vi "initialize assembly lists.vi"(4 "output dictionary":refnum<class "data dictionary.lvclass">, 6 "input dictionary":refnum<class "data dictionary.lvclass">, 8 "error in":errorcluster, 10 "EthernetIP configuration in":refnum<class "EthernetIP configuration.lvclass">, 11 "EthernetIP runtime in":refnum<class "EthernetIP runtime.lvclass">) -> (0 "error out":errorcluster, 3 "EthernetIP runtime out":refnum<class "EthernetIP runtime.lvclass">)   [LabVIEW 2013, in "EthernetIP runtime.lvclass"]
uses:
  EthernetIP runtime.lvclass
  configuration/EthernetIP configuration.lvclass
  <vilib>/NI/Tag Bus/dictionary/data dictionary.lvclass
  <vilib>/ethernetip/ethernetip.llb/ethernetip.ctl
  assembly data spec.ctl
  conversion specification.ctl
  <vilib>/NI/Tag Bus/tag/Data Type.ctl
  configuration/EthernetIP configuration.lvclass/EthernetIP configuration.ctl
  <vilib>/ethernetip/ethernetip.llb/EthernetIPAssemblyType.ctl
  channel/EthernetIP Channel.lvclass/EthernetIP Channel.ctl
  <vilib>/NI/Tag Bus/tag/tag descriptor.lvclass/tag descriptor.ctl
  <vilib>/NI/Tag Bus Module Framework/channel/TBM channel.lvclass/TBM channel.ctl
  EthernetIP runtime.lvclass/EthernetIP runtime.ctl
  channel/Read Instance ID.vi
  <vilib>/NI/Tag Bus/tag/read tag name.vi
  <vilib>/NI/Tag Bus Module Framework/channel/Read channel classification.vi
  <vilib>/NI/Tag Bus/tag/read data type.vi
  channel/Read byte index.vi
  configuration/Read assemblies.vi
  configuration/read eip channels.vi
  channel/EthernetIP Channel.lvclass
  <vilib>/NI/Tag Bus/tag/tag descriptor.lvclass
  <vilib>/ethernetip/ethernetip.lvlib
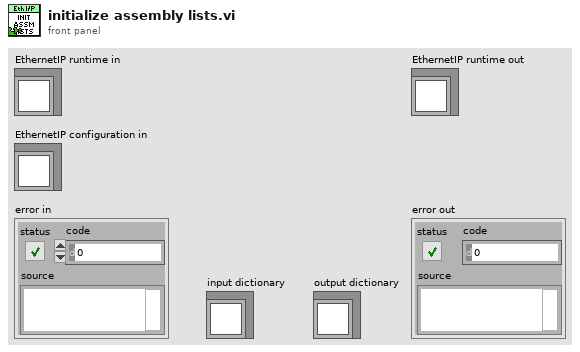
[diagram p1: front panel]
types:
  T1 = typedef "EthernetIP runtime.lvclass/assembly data spec.ctl" = cluster{"Instance ID":u32, "specification":T2[], "big endian?":bool}
  T2 = typedef "EthernetIP runtime.lvclass/conversion specification.ctl" = cluster{"data type":T3, "data index":i32, "byte index":i32, "subindex/len":i32}
  T3 = typedef "tag bus.lvlib/tag descriptor.lvclass/Data Type.ctl" = enum16{"Double", "Single", "I64", "I32", "I16", "I8", "U64", "U32", "U16", "U8", "Boolean", "String", "Array of Double", "Array of Single", "Array of I64", "Array of I32", "Array of I16", "Array of I8", "Array of U64", "Array of U32", "Array of U16", "Array of U8", "Array of Boolean", "Array of String"}
  T4 = typedef "ethernetip.lvlib/ethernetip.ctl" = refnum<k21>
  T5 = typedef "EthernetIP configuration.lvclass/assembly definition.ctl" = cluster{"name":string, "Instance ID":u32, "Type":T6, "Size (elements)":u32, "big endian?":bool, "data type":T3}
  T6 = typedef "EthernetIP configuration.lvclass/assembly type.ctl" = enum32{"Producing", "Consuming"}
  T7 = typedef "ethernetip.lvlib/EthernetIPAssemblyType.ctl" = enum16{"Producing", "Consuming", "Configuration"}
  T8 = typedef "TBM channel.lvclass/channel classification.ctl" = enum16{"input data", "output data", "processing parameter", "processing result"}
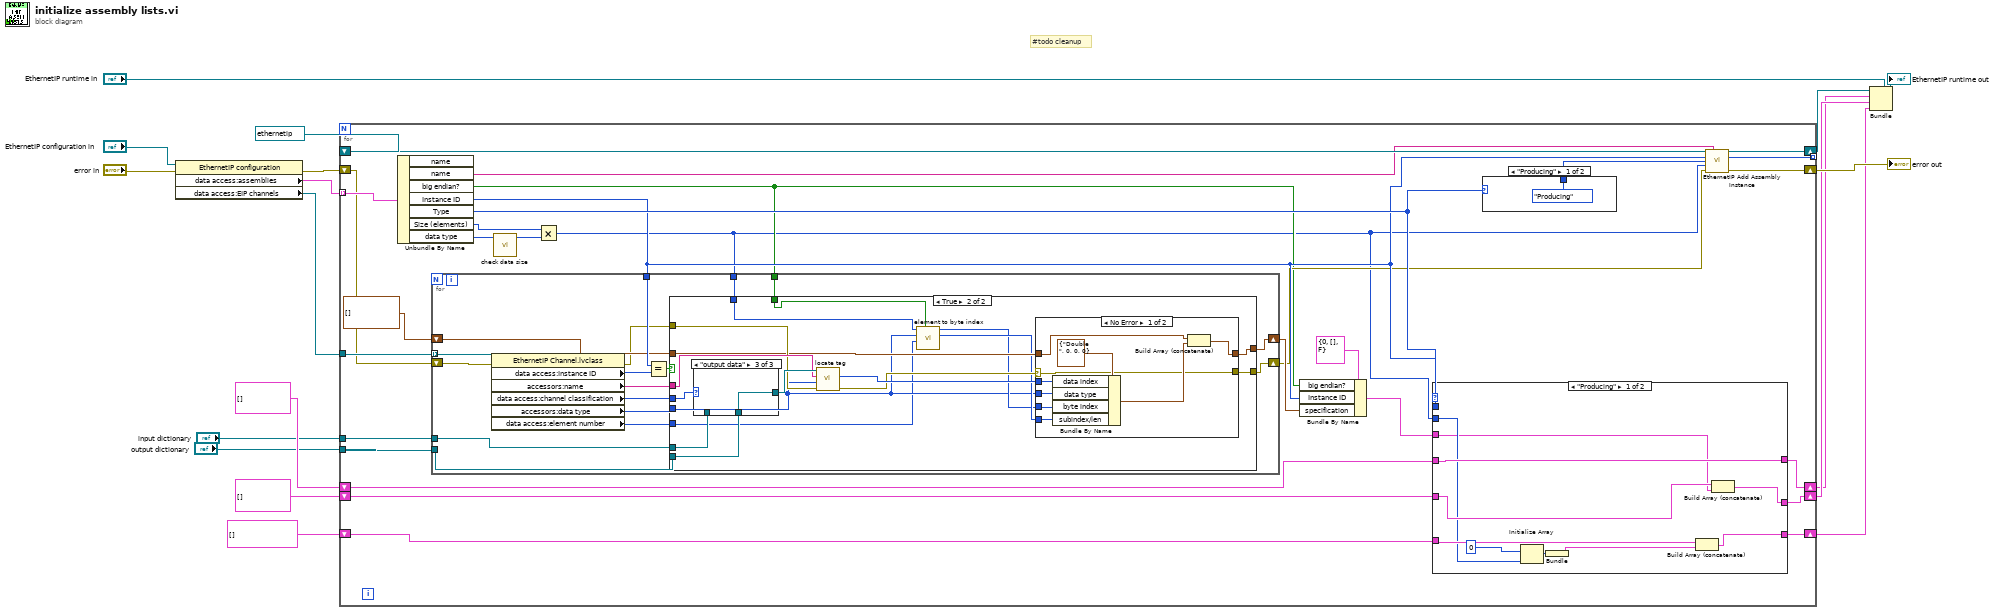
[diagram p0: block diagram]
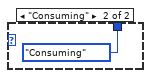
[diagram p6: hidden frame]
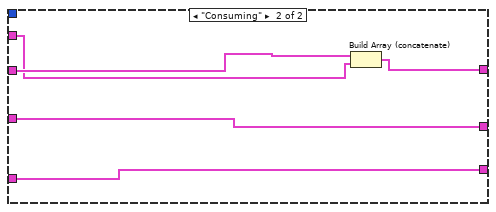
[diagram p7: hidden frame]
diagram:
  # "#todo cleanup"
  n1 = property class="EthernetIP configuration"(reference="EthernetIP configuration in", error in="error in") -> (error out=w14:errorcluster, "data access:assemblies"=w17:T5[], "data access:EIP channels"=w18:refnum<class "EthernetIP Channel.lvclass">[])  [unwired: 1 out]
  n2 = for {
    shift-right: [w47] -> w11
    shift-left: w14 -> [w27]
    shift-right: [w46] -> w13
    shift-left: T4 "Default" ("Session in") -> [w45]
    tunnel: w17 -> [w44] mode=indexing
    tunnel: [w42] -> _ mode=indexing
    tunnel: w18 -> [w33]
    shift-right: [w34] -> w3
    shift-left: T1[] [] ("output assemblies") -> [w35]
    shift-right: [w39] -> w4
    shift-left: T1[] [] ("output assemblies") -> [w38]
    shift-right: [w36] -> w5
    shift-left: cluster{"output allocation":u8[]}[] [] ("output allocations") -> [w37]
    tunnel: "input dictionary" -> [w25]
    tunnel: "output dictionary" -> [w24]
    n3 = Unbundle By Name(w44) -> ("name"=w43:string, "big endian?"=w23:bool, "Instance ID"=w30:u32, "Type"=w41:T6, "Size (elements)"=w20:u32, "data type"=w22:T3)  [unwired: 1 out]
    n4 = call "check data size.vi"("data type"=w22) -> ("bytes"=w21:i32)  [unwired: 10 in]
    n5 = Multiply(x=w20, y=w21) -> (x*y=w19:u32)
    n6 = for {
      tunnel: w33 -> [w64] mode=indexing
      tunnel: w30 -> [w63]
      shift-right: [w62] -> w29
      shift-left: T2[] [] ("specification") -> [w61]
      shift-right: [w50] -> w26
      shift-left: w27 -> [w56]
      tunnel: w25 -> [w54]
      tunnel: w24 -> [w53]
      tunnel: w23 -> [w49]
      tunnel: w19 -> [w48]
      n7 = property class="EthernetIP Channel.lvclass"(reference=w64, error in=w56) -> (error out=w51:errorcluster, "data access:Instance ID"=w57:u32, "accessors:name"=w52:string, "data access:channel classification"=w55:T8, "accessors:data type"=w58:T3, "data access:element number"=w59:i32)  [unwired: 1 out]
      n8 = Equal?(x=w63, y=w57) -> (x = y?=w60:bool)
      n9 = case shown="True" w60 {
        tunnel: [w66 w83] -> w62
        tunnel: w61 -> [w66 w73]
        tunnel: w59 -> [_ w68]
        tunnel: w58 -> [_ w69]
        tunnel: w55 -> [_ w82]
        tunnel: w54 -> [_ w81]
        tunnel: w53 -> [_ w80]
        tunnel: w52 -> [_ w78]
        tunnel: w51 -> [w65 w77]
        tunnel: [w65 w74] -> w50
        tunnel: w49 -> [_ w70]
        tunnel: w48 -> [_ w67]
        frame False {
        }
        frame True {
          n10 = case shown="\"output data\"" w82 {
            tunnel: w81 -> [w84 _ _]
            tunnel: w80 -> [_ _ w85]
            tunnel: [w84 _ w85] -> w79
            frame "input data" {
            }
            frame Default {
            }
            frame "output data" {
            }
          }
          n11 = call <vilib>:"locate tag.vi"("error in"=w77, "data type"=w69, "name"=w78, "data dictionary in"=w79) -> ("error out"=w75:errorcluster, "index"=w76:i32)  [unwired: 5 in, 1 out]
          n12 = call "element to byte index.vi"("big endian?"=w70, "element number"=w68, "data type"=w69, "assembly size (bytes)"=w67) -> ("subindex"=w72:i32, "byte index"=w71:i32)  [unwired: 6 in]
          n13 = case shown="No Error" w75 {
            selector: w75 -> [w87 w95]
            tunnel: [w89 w96] -> w83
            tunnel: w73 -> [w90 w96]
            tunnel: w71 -> [w93 _]
            tunnel: w69 -> [w92 _]
            tunnel: w76 -> [w88 _]
            tunnel: [w87 w95] -> w74
            tunnel: w72 -> [w86 _]
            frame No Error {
              n14 = Bundle By Name(cluster=T2 {"data type"=enum."Double", "data index"=0, "byte index"=0, "subindex/len"=0} ("specification"), "data index"=w88, "data type"=w92, "byte index"=w93, "subindex/len"=w86) -> (w91:T2)
              n15 = Build Array (concatenate)(w90, w91) -> (w89:T2[])
            }
            frame Error {
            }
          }
        }
      }
    }
    n16 = Bundle By Name(cluster=T1 {"Instance ID"=0, "specification"=[], "big endian?"=FALSE} ("assembly data spec"), "big endian?"=w23, "Instance ID"=w30, "specification"=w29) -> (w28:T1)
    n17 = case shown="\"Producing\"" w41 {
      tunnel: w30 -> [_ _]
      tunnel: w19 -> [w103 _]
      tunnel: [w108 w113] -> w39
      tunnel: w38 -> [w107 w113]
      tunnel: w37 -> [w105 w112]
      tunnel: [w106 w112] -> w36
      tunnel: w35 -> [w104 w111]
      tunnel: [w104 w110] -> w34
      tunnel: w28 -> [w99 w109]
      frame "Producing" {
        n18 = Initialize Array(u8 0, w103) -> (w101:u8[])
        n19 = Bundle(w101) -> (w100:cluster{u8[]})  [unwired: 1 in]
        n20 = Build Array (concatenate)(w105, w100) -> (w106:cluster{"output allocation":u8[]}[])
        n21 = Build Array (concatenate)(w107, w99) -> (w108:T1[])
      }
      frame "Consuming" {
        n22 = Build Array (concatenate)(w111, w109) -> (w110:T1[])
      }
    }
    n23 = case shown="\"Producing\"" w41 {
      tunnel: [EthernetIPAssemblyType."Producing" ("Type") EthernetIPAssemblyType."Consuming" ("Type")] -> w40
      frame "Producing" {
      }
      frame "Consuming" {
      }
    }
    n24 = call <vilib>:"EthernetIP Add Assembly Instance.vi"("Session in"=w45, "Name (optional)"=w43, "Instance ID in"=w30, "Type"=w40, "Size (bytes)"=w19, "error in"=w26) -> ("Session out"=w46:T4, "Instance ID out"=w42:u32, "error out"=w47:errorcluster)  [unwired: 7 in]
  }
  "error out" <- w11
  n25 = Bundle(cluster="EthernetIP runtime in", w13, w3, w4, w5) -> (→"EthernetIP runtime out":refnum<class "EthernetIP runtime.lvclass">)
